vi "PRIME Set Mode.vi"(8 "error in (no error)":errorcluster, 10 "Integration Mode":T1, 11 "connection ID":refnum<k5>) -> (0 "error out":errorcluster, 2 "Command":string, 3 "connection ID out":refnum<k5>)   [LabVIEW 2021, in "PRIME Detector.lvclass"]
uses:
  PRIME Detector.lvclass
  Detector enum Detector Integration Mode.ctl
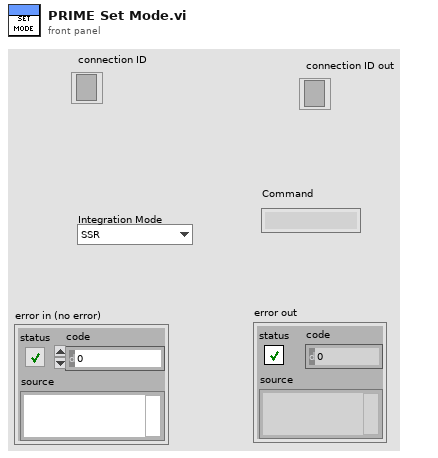
[diagram p1: front panel]
types:
  T1 = typedef "Detector enum Detector Integration Mode.ctl" = enum16{"SSR", "CDS", "MEAN", "MEDIAN", "MODE", "MIIN", "MAX"}
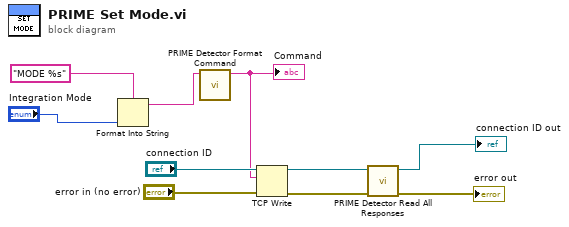
[diagram p0: block diagram]
diagram:
  n1 = Format Into String(format string="MODE %s" ("Command"), "Integration Mode") -> (resulting string=w2:string)  [unwired: 2 in, 1 out]
  n2 = call "PRIME Detector Format Command.vi"("Command"=w2) -> ("TCP String"=w5:string)  [unwired: 10 in]
  "Command" <- w5
  n3 = TCP Write(connection ID="connection ID", data in=w5, error in (no error)="error in (no error)") -> (connection ID out=w8:refnum<k5>, error out=w7:errorcluster)  [unwired: 1 in, 1 out]
  n4 = call "PRIME Detector Read All Responses.vi"("error in"=w7, "connection ID"=w8) -> ("error out"=→"error out":errorcluster, "connection ID out"=→"connection ID out":refnum<k5>)  [unwired: 6 in, 2 out]
